vi "HEWH Power Notifier.vi"(7 "Status":T2, 8 "error in (no error)":errorcluster, 10 "Set Status":T1, 11 "name (unnamed)":string) -> (0 "error out":errorcluster, 3 "latest notification":T1)   [LabVIEW 2016]
uses:
  Utility/Type Definitions/UTILITY Notifier.ctl
  Type Definitions/HEWH Power Elements.ctl
panel:
  in  "POWER (Data Type)":T1
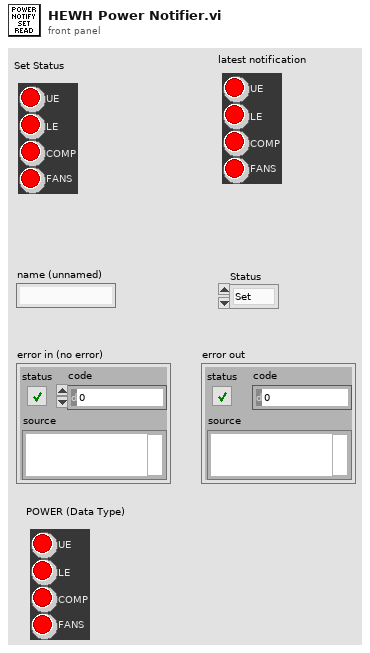
[diagram p1: front panel]
types:
  T1 = typedef "HEWH Power Elements.ctl" = cluster{"UE":bool, "LE":bool, "COMP":bool, "FANS":bool}
  T2 = typedef "UTILITY Notifier.ctl" = enum16{"Set", "Read", "Release Ref"}
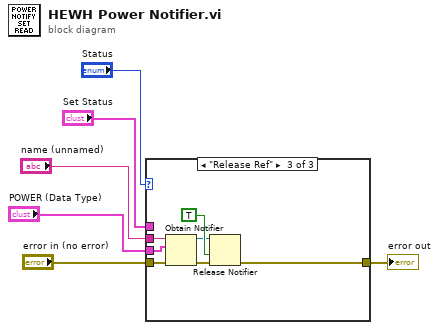
[diagram p0: block diagram]
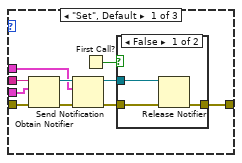
[diagram p2: hidden frame]
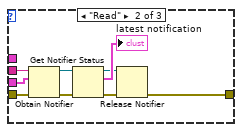
[diagram p4: hidden frame]
diagram:
  n1 = case shown="\"Release Ref\"" "Status" {
    tunnel: [w7 w22 w32] -> w6
    tunnel: "error in (no error)" -> [w14 w27 w33]
    tunnel: "name (unnamed)" -> [w13 w26 w31]
    tunnel: "POWER (Data Type)" -> [w11 w25 w30]
    tunnel: "Set Status" -> [w12 _ _]
    frame "Set", Default {
      n2 = Obtain Notifier(name (unnamed)=w13, notification data type=w11, error in (no error)=w14) -> (notifier out=w15:refnum<notifier>, error out=w16:errorcluster)  [unwired: 1 in, 1 out]
      n3 = Send Notification(notification=w12, notifier=w15, error in (no error)=w16) -> (notifier out=w9:refnum<notifier>, error out=w10:errorcluster)
      n4 = First Call?() -> (First Call?: T/F=w8:bool)
      n5 = case shown="False" w8 {
        tunnel: w10 -> [w19 w20]
        tunnel: [w18 w20] -> w7
        tunnel: w9 -> [w17 _]
        frame False {
          n6 = Release Notifier(notifier=w17, error in (no error)=w19) -> (error out=w18:errorcluster)  [unwired: 1 in, 2 out]
        }
        frame True {
        }
      }
    }
    frame "Read" {
      n7 = Obtain Notifier(name (unnamed)=w26, notification data type=w25, error in (no error)=w27) -> (notifier out=w28:refnum<notifier>, error out=w29:errorcluster)  [unwired: 1 in, 1 out]
      n8 = Get Notifier Status(notifier=w28, error in (no error)=w29) -> (notifier out=w21:refnum<notifier>, current notification=→"latest notification":T1, error out=w23:errorcluster)  [unwired: 2 out]
      n9 = Release Notifier(notifier=w21, error in (no error)=w23) -> (error out=w22:errorcluster)  [unwired: 1 in, 2 out]
    }
    frame "Release Ref" {
      n10 = Obtain Notifier(name (unnamed)=w31, notification data type=w30, error in (no error)=w33) -> (notifier out=w35:refnum<notifier>, error out=w34:errorcluster)  [unwired: 1 in, 1 out]
      n11 = Release Notifier(notifier=w35, force destroy? (F)=TRUE, error in (no error)=w34) -> (error out=w32:errorcluster)  [unwired: 2 out]
    }
  }
  "error out" <- w6
